vi "Increment Error Counts.vi"(4 "specific errors":T3, 6 "receiving errors":i16, 8 "error in":errorcluster, 11 "status error channel data references":T2 {"receiving" format="%.0x"; "specific errors"."gap" format="%.0x"; "specific errors"."parity" format="%.0x"; "specific errors"."long word" format="%.0x"; "specific errors"."bit timing" format="%.0x"; "specific errors"."timeout" format="%.0x"}) -> (0 "error out":errorcluster)   [LabVIEW 2020, in "Ballard ARINC 429 Engine.lvlib" / "Implementation.lvlib" / "Ballard ARINC-429 Rx Execution Unit.lvclass"]
uses:
  Ballard ARINC-429 Rx Execution Unit.lvclass
  <vilib>/NI VeriStand/Custom Device API/Custom Device API.lvlib
  <vilib>/NI VeriStand/Custom Device API/Data Reference.ctl
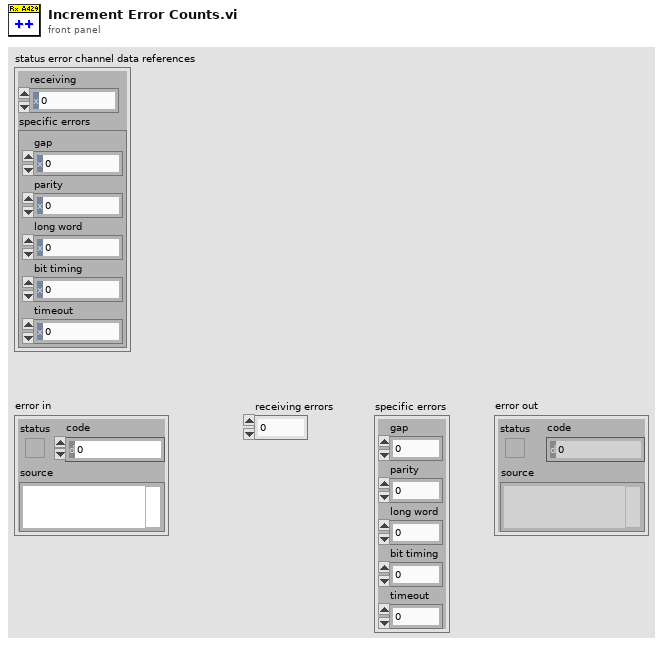
[diagram p1: front panel]
types:
  T1 = typedef "Custom Device API.lvlib/Data Reference.ctl" = i32
  T2 = cluster{"receiving":T1, "specific errors":cluster{"gap":T1, "parity":T1, "long word ":T1, "bit timing":T1, "timeout":T1}}
  T3 = cluster{"gap":i16, "parity":i16, "long word":i16, "bit timing":i16, "timeout":i16}
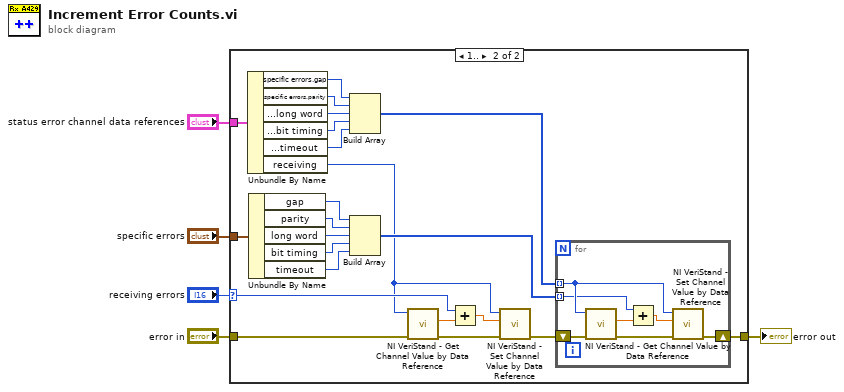
[diagram p0: block diagram]
diagram:
  n1 = case shown="1.." "receiving errors" {
    selector: "receiving errors" -> [_ w22]
    tunnel: [w6 w28] -> w5
    tunnel: "status error channel data references" -> [_ w26]
    tunnel: "specific errors" -> [_ w24]
    tunnel: "error in" -> [w6 w7]
    frame Default {
    }
    frame 1.. {
      n2 = Unbundle By Name(w26) -> ("specific errors.gap"=w20:T1, "specific errors.parity"=w19:T1, "specific errors.long word"=w18:T1, "specific errors.bit timing"=w17:T1, "specific errors.timeout"=w16:T1, "receiving"=w8:T1)
      n3 = Unbundle By Name(w24) -> ("gap"=w12:i16, "parity"=w14:i16, "long word"=w15:i16, "bit timing"=w13:i16, "timeout"=w11:i16)
      n4 = Build Array(w20, w19, w18, w17, w16) -> (w10:T1[])
      n5 = Build Array(w12, w14, w15, w13, w11) -> (w9:i16[])
      n6 = call <vilib>:"NI VeriStand - Get Channel Value by Data Reference.vi"("error in (no error)"=w7, "Data Reference in"=w8) -> ("error out"=w27:errorcluster, "Value"=w23:dbl)  [unwired: 8 in]
      n7 = Add(x=w22, y=w23) -> (x+y=w21:dbl)
      n8 = call <vilib>:"NI VeriStand - Set Channel Value by Data Reference.vi"("error in (no error)"=w27, "Value"=w21, "Data Reference in"=w8) -> ("error out"=w25:errorcluster)  [unwired: 8 in]
      n9 = for {
        shift-right: [w34] -> w28
        shift-left: w25 -> [w33]
        tunnel: w10 -> [w32] mode=indexing
        tunnel: w9 -> [w29] mode=indexing
        n10 = call <vilib>:"NI VeriStand - Get Channel Value by Data Reference.vi"("error in (no error)"=w33, "Data Reference in"=w32) -> ("error out"=w35:errorcluster, "Value"=w31:dbl)  [unwired: 8 in]
        n11 = Add(x=w29, y=w31) -> (x+y=w30:dbl)
        n12 = call <vilib>:"NI VeriStand - Set Channel Value by Data Reference.vi"("error in (no error)"=w35, "Value"=w30, "Data Reference in"=w32) -> ("error out"=w34:errorcluster)  [unwired: 8 in]
      }
    }
  }
  "error out" <- w5
